vi "Open products FP in SP.vi"(8 "error in (no error)":errorcluster, 11 "Productos in":refnum<class "Productos.lvclass">) -> (0 "error out":errorcluster, 3 "Productos out":refnum<class "Productos.lvclass">)   [LabVIEW 2020, in "Productos.lvlib" / "Productos.lvclass"]
uses:
  Productos.lvclass
  Productos.lvclass/Productos.ctl
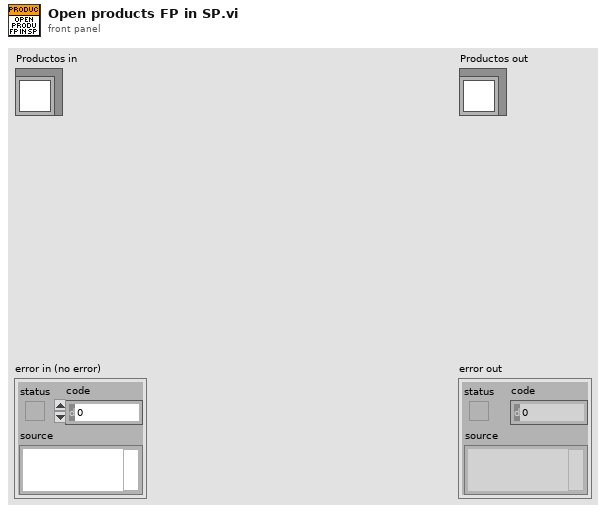
[diagram p1: front panel]
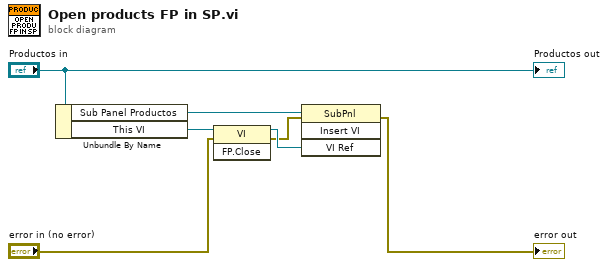
[diagram p0: block diagram]
diagram:
  n1 = Unbundle By Name("Productos in") -> ("Sub Panel Productos"=w6:refnum<vi>, "This VI"=w4:refnum<vi>)
  n2 = invoke class="VI" method="FP.Close"(reference=w4, error in="error in (no error)") -> (reference out=w5:refnum<vi>, error out=w3:errorcluster)  [unwired: 1 in, 1 out]
  n3 = invoke class="SubPnl" method="Insert VI"(reference=w6, error in=w3, "VI Ref"=w5) -> (error out=→"error out":errorcluster)  [unwired: 1 in, 3 out]
  "Productos out" <- "Productos in"
